vi "PSVCH_Convert Data.vi"(10 "InUsedModu[]":T2(array[cluster])) -> (2 "VarList":cluster{"Tag":string[], "Name":string[]})   [LabVIEW 2016]
uses:
  HardWare/Ctrls/HardWare _ Channel Parameters.ctl
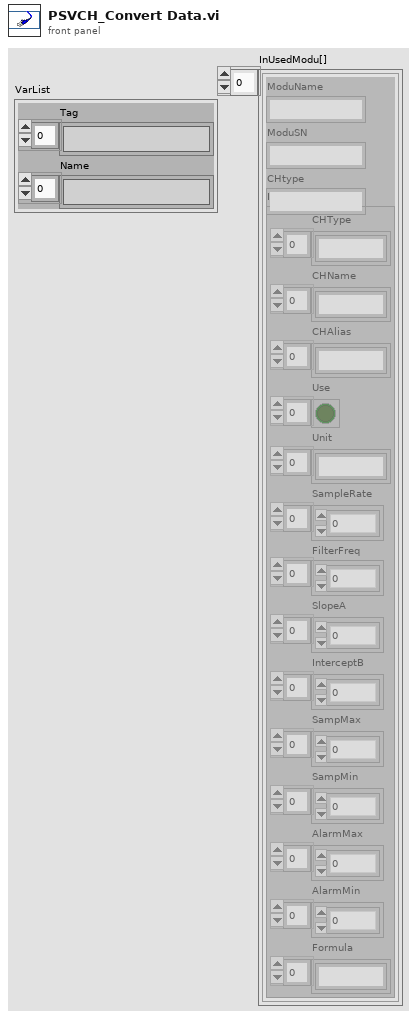
[diagram p1: front panel]
types:
  T1 = typedef "HardWare _ Channel Parameters.ctl" = cluster{"CHType":string[], "CHName":string[], "CHAlias":string[], "Use":bool[], "Unit":string[], "SampleRate":dbl[], "FilterFreq":dbl[], "SlopeA":dbl[], "InterceptB":dbl[], "SampMax":dbl[], "SampMin":dbl[], "AlarmMax":dbl[], "AlarmMin":dbl[], "Formula":string[]}
  T2 = cluster{"ModuName":string, "ModuSN":string, "CHtype":string, "InUsedChanPara[]":T1}[]
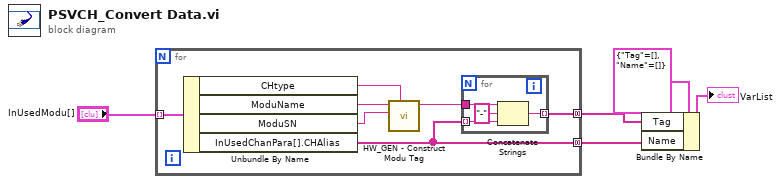
[diagram p0: block diagram]
diagram:
  n1 = for {
    tunnel: [w10] -> w4 mode=concatenating
    tunnel: [w11] -> w3 mode=concatenating
    tunnel: "InUsedModu[]" -> [w12] mode=indexing
    n2 = Unbundle By Name(w12) -> ("CHtype"=w7:string, "ModuName"=w9:string, "ModuSN"=w8:string, "InUsedChanPara[].CHAlias"=w11:string[])
    n3 = call "HW_GEN - Construct Modu Tag.vi"("ChanType"=w7, "ModSN"=w8, "ModName"=w9) -> ("String"=w6:string)  [unwired: 8 in]
    n4 = for {
      tunnel: w6 -> [w16]
      tunnel: w11 -> [w15] mode=indexing
      tunnel: [w13] -> w10 mode=indexing
      n5 = Concatenate Strings(w16, "-" ("string"), w15) -> (w13:string)
    }
  }
  n6 = Bundle By Name(cluster=cluster{"Tag":string[], "Name":string[]} {"Tag"=[], "Name"=[]} ("VarList"), "Tag"=w4, "Name"=w3) -> (→"VarList":cluster{"Tag":string[], "Name":string[]})
